vi "ArmSimulator.vi"() -> ()   [LabVIEW 2020]
uses:
  <vilib>/robotics/Kinematics/DH Kinematic Parameters.ctl
  <vilib>/robotics/Kinematics/Link/Joint Type.ctl
  <vilib>/Utility/miscctls.llb/LV3DPointTypeDef.ctl
  de8be538-574b-4146-99e0-83cb54bb3f19.vi
  a5137bdd-6b26-409e-be81-2a36b3426dbb.vi
  <vilib>/robotics/Kinematics/RotateX.vi
  <vilib>/robotics/Kinematics/RotateY.vi
  <vilib>/robotics/Kinematics/RotateZ.vi
  <vilib>/Analysis/baseanly.llb/A x B.vi
  <vilib>/Analysis/baseanly.llb/Real A x B.vi
  <vilib>/robotics/Kinematics/Analytical/Initialize Generic Serial Arm.vi
  <vilib>/robotics/Kinematics/Robot/Forward Kinematics (Point).vi
  <vilib>/picture/3D Picture Control/Object/Create Object (drawable).vi
  <vilib>/Analysis/Matrix/Comparison/Not Equal/Not Equal.vi
  <vilib>/Analysis/Matrix/Comparison/Not Equal/Not Equal - RM,RM.vi
  <vilib>/picture/3D Picture Control/Object/Add Object (no reference).vi
  <vilib>/robotics/Kinematics/Analytical/NI_Robotics_AnalyticKinematics.lvlib
  <vilib>/robotics/Kinematics/Link/NI_Robotics_Link.lvclass
  <vilib>/robotics/Kinematics/Robot/NI_Robotics_Serial Robot Arm.lvclass
  <vilib>/robotics/Kinematics/Plotting/NI_Robotics_3DKinematics.lvlib
  <vilib>/picture/3D Picture Control/NI_3D Picture Control.lvlib
  <vilib>/robotics/Kinematics/NI_Kinematics.lvlib
panel:
  in  "Wrist Position":bool
  out "Steps Taken":i32
  in  "Reset 3D View":bool
  out "IK Error":errorcluster
  in  "Goal Z (in)":dbl=28.0
  in  "Goal X (in)":dbl=-33.0
  out "3D Arm Simulation":refnum<vi>(3d-picture)
  # "<-- DOWN FIELD              SCORING GRID -->"
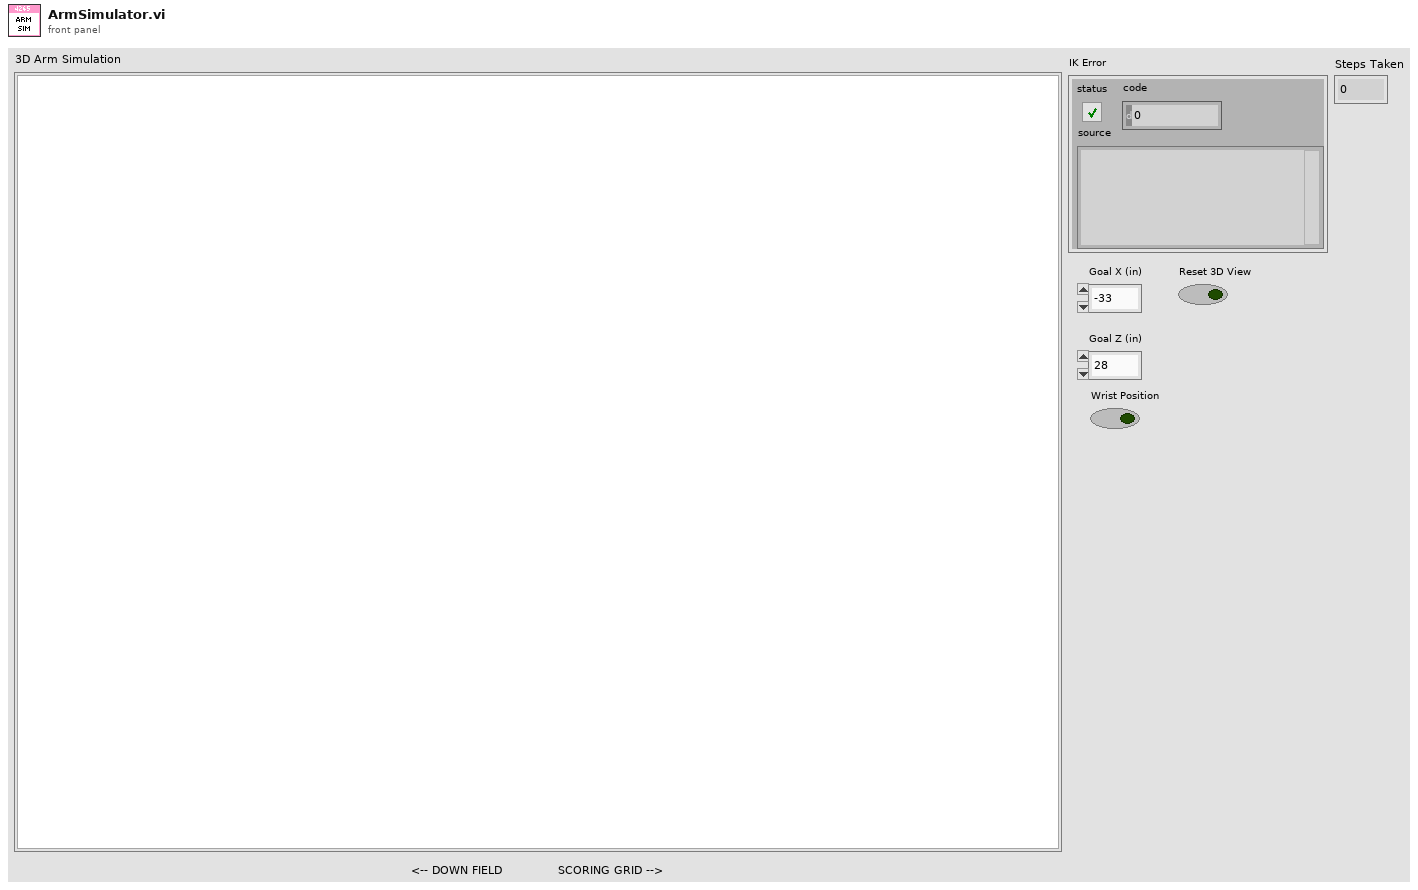
[diagram p1: front panel]
types:
  T1 = typedef "DH Kinematic Parameters.ctl" = cluster{"twist angle":dbl, "length":dbl, "rotation angle":dbl, "offset distance":dbl, "joint type":T2, "joint coordinate offset":dbl}
  T2 = typedef "NI_Robotics_Link.lvclass/Joint Type.ctl" = enum16{"Revolute", "Prismatic"}
  T3 = typedef "NI_Matrix.lvlib/RealMatrix.ctl" = dbl[][]
  T4 = cluster{"Red":sgl, "Green":sgl, "Blue":sgl, "Alpha":sgl}
  T5 = typedef "LV3DPointTypeDef.ctl" = cluster{"X":sgl, "Y":sgl, "Z":sgl}
  T6 = cluster{"Goal X (in)":dbl, "Goal Y (in)":dbl, "Goal Z (in)":dbl}
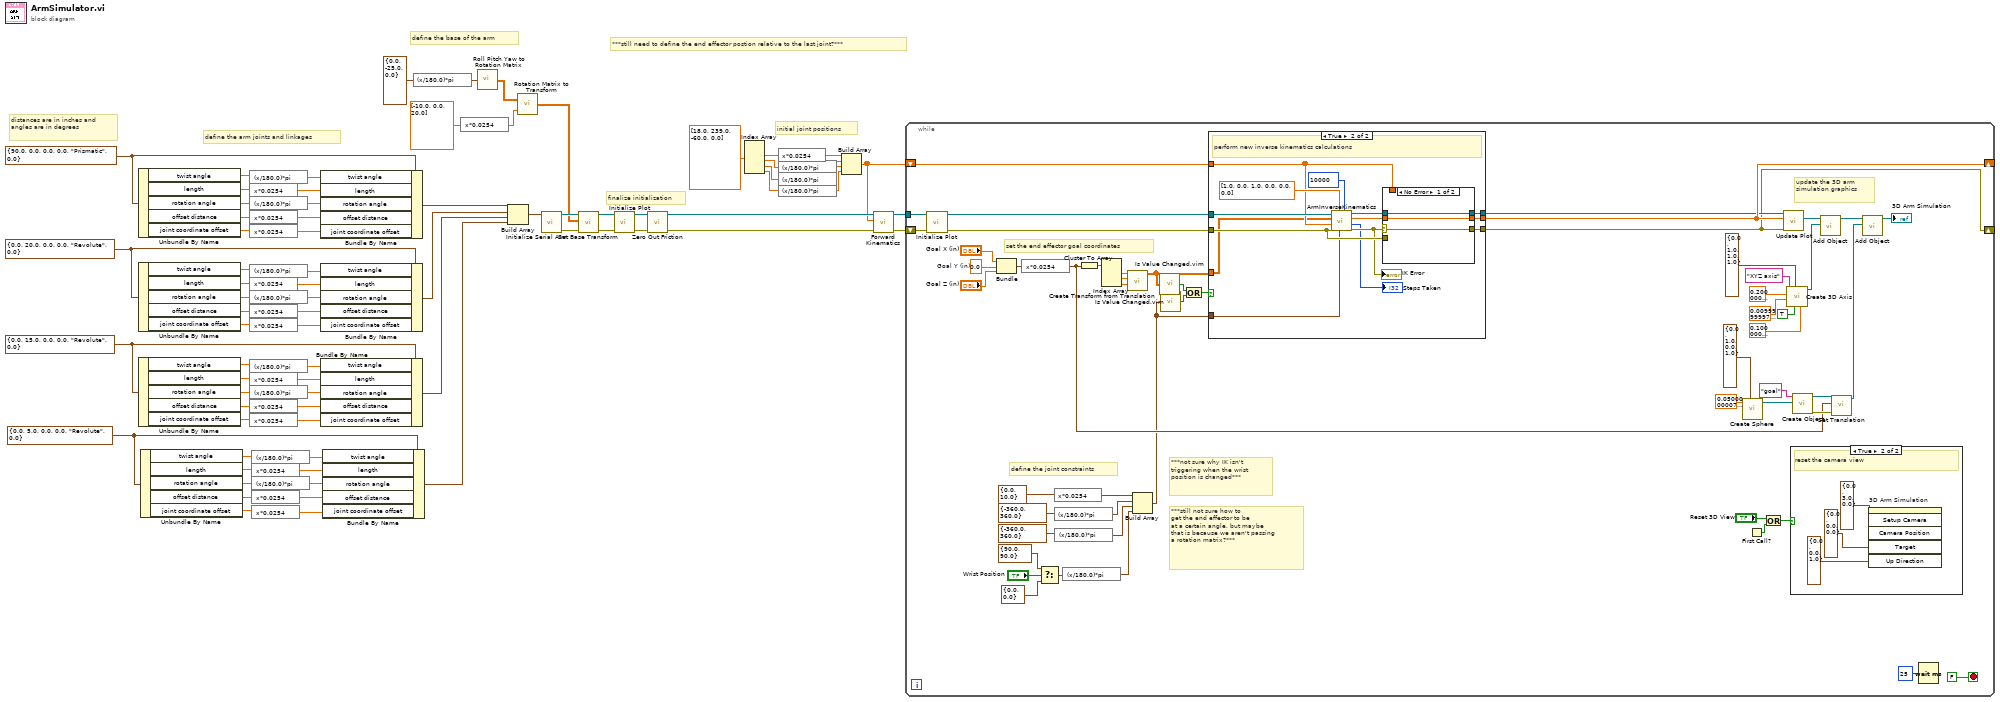
[diagram p0: block diagram]
diagram:
  w13 = T1 {"twist angle"=0.0, "length"=5.0, "rotation angle"=0.0, "offset distance"=0.0, "joint type"=enum."Revolute", "joint coordinate offset"=0.0} ("Link Parameters")
  w49 = T1 {"twist angle"=0.0, "length"=15.0, "rotation angle"=0.0, "offset distance"=0.0, "joint type"=enum."Revolute", "joint coordinate offset"=0.0} ("Link Parameters")
  w60 = T1 {"twist angle"=0.0, "length"=20.0, "rotation angle"=0.0, "offset distance"=0.0, "joint type"=enum."Revolute", "joint coordinate offset"=0.0} ("Link Parameters")
  w72 = T1 {"twist angle"=90.0, "length"=0.0, "rotation angle"=0.0, "offset distance"=0.0, "joint type"=enum."Prismatic", "joint coordinate offset"=0.0} ("Link Parameters")
  # "***still need to define the end effector postion relative to the last joint?***"
  # "initial joint positions"
  # "define the arm joints and linkages"
  # "define the base of the arm"
  # "distances are in inches and\nangles are in degrees"
  # "finalize initialization"
  n1 = Unbundle By Name(w72) -> ("twist angle"=w71:dbl, "length"=w67:dbl, "rotation angle"=w69:dbl, "offset distance"=w65:dbl, "joint coordinate offset"=w63:dbl)
  n2 = Unbundle By Name(w60) -> ("twist angle"=w59:dbl, "length"=w56:dbl, "rotation angle"=w58:dbl, "offset distance"=w54:dbl, "joint coordinate offset"=w52:dbl)
  n3 = Unbundle By Name(w49) -> ("twist angle"=w48:dbl, "length"=w45:dbl, "rotation angle"=w47:dbl, "offset distance"=w43:dbl, "joint coordinate offset"=w41:dbl)
  n4 = Unbundle By Name(w13) -> ("twist angle"=w12:dbl, "length"=w9:dbl, "rotation angle"=w11:dbl, "offset distance"=w7:dbl, "joint coordinate offset"=w5:dbl)
  n5 = expression code="(x/180.0)*pi" ("degrees to radians")(w71) -> (w73:dbl)
  n6 = expression code="x*0.0254" ("degrees to radians")(w67) -> (w66:dbl)
  n7 = expression code="(x/180.0)*pi" ("degrees to radians")(w69) -> (w68:dbl)
  n8 = expression code="x*0.0254" ("degrees to radians")(w65) -> (w64:dbl)
  n9 = expression code="x*0.0254" ("degrees to radians")(w63) -> (w62:dbl)
  n10 = expression code="(x/180.0)*pi" ("degrees to radians")(w59) -> (w61:dbl)
  n11 = expression code="x*0.0254" ("degrees to radians")(w56) -> (w55:dbl)
  n12 = expression code="(x/180.0)*pi" ("degrees to radians")(w58) -> (w57:dbl)
  n13 = expression code="x*0.0254" ("degrees to radians")(w54) -> (w53:dbl)
  n14 = expression code="x*0.0254" ("degrees to radians")(w52) -> (w51:dbl)
  n15 = expression code="(x/180.0)*pi" ("degrees to radians")(w48) -> (w50:dbl)
  n16 = expression code="x*0.0254" ("degrees to radians")(w45) -> (w44:dbl)
  n17 = expression code="(x/180.0)*pi" ("degrees to radians")(w47) -> (w46:dbl)
  n18 = expression code="x*0.0254" ("degrees to radians")(w43) -> (w42:dbl)
  n19 = expression code="x*0.0254" ("degrees to radians")(w41) -> (w40:dbl)
  n20 = expression code="(x/180.0)*pi" ("degrees to radians")(w12) -> (w14:dbl)
  n21 = expression code="x*0.0254" ("degrees to radians")(w9) -> (w8:dbl)
  n22 = expression code="(x/180.0)*pi" ("degrees to radians")(w11) -> (w10:dbl)
  n23 = expression code="x*0.0254" ("degrees to radians")(w7) -> (w6:dbl)
  n24 = expression code="x*0.0254" ("degrees to radians")(w5) -> (w4:dbl)
  n25 = Bundle By Name(cluster=w72, "twist angle"=w73, "length"=w66, "rotation angle"=w68, "offset distance"=w64, "joint coordinate offset"=w62) -> (w70:T1)
  n26 = Bundle By Name(cluster=w60, "twist angle"=w61, "length"=w55, "rotation angle"=w57, "offset distance"=w53, "joint coordinate offset"=w51) -> (w39:T1)
  n27 = Bundle By Name(cluster=w49, "twist angle"=w50, "length"=w44, "rotation angle"=w46, "offset distance"=w42, "joint coordinate offset"=w40) -> (w38:T1)
  n28 = Bundle By Name(cluster=w13, "twist angle"=w14, "length"=w8, "rotation angle"=w10, "offset distance"=w6, "joint coordinate offset"=w4) -> (w3:T1)
  n29 = expression code="(x/180.0)*pi" ("degrees to radians")(cluster{"roll":dbl, "pitch":dbl, "yaw":dbl} {"roll"=0.0, "pitch"=-25.0, "yaw"=0.0} ("angles")) -> (w33:cluster{"roll":dbl, "pitch":dbl, "yaw":dbl})
  n30 = expression code="x*0.0254" ("degrees to radians")(dbl[] [-10.0, 0.0, 20.0] ("translation vector")) -> (w28:dbl[])
  n31 = call <vilib>:"Roll Pitch Yaw to Rotation Matrix.vi"("angles"=w33) -> ("rotation matrix"=w35:T3)
  n32 = Build Array(w70, w39, w38, w3) -> (w37:T1[])
  n33 = call <vilib>:"Rotation Matrix to Transform.vi"("translation vector"=w28, "rotation matrix"=w35) -> ("transform"=w32:T3)
  n34 = call-poly <vilib>:"Initialize Serial Arm.vi"("kinematic parameters"=w37) -> ("error out"=w30:errorcluster, "serial arm out"=w36:refnum<class "NI_Robotics_Serial Robot Arm.lvclass">)  [unwired: 9 in]
  n35 = call <vilib>:"Set Base Transform.vi"("error in (no error)"=w30, "base transform"=w32, "serial arm in"=w36) -> ("error out"=w29:errorcluster, "serial arm out"=w31:refnum<class "NI_Robotics_Serial Robot Arm.lvclass">)  [unwired: 7 in]
  n36 = call <vilib>:"Initialize Plot.vi"("error in (no error)"=w29, "serial arm in"=w31) -> ("error out"=w75:errorcluster, "serial arm out"=w74:refnum<class "NI_Robotics_Serial Robot Arm.lvclass">)  [unwired: 8 in]
  n37 = call <vilib>:"Zero Out Friction.vi"("error in (no error)"=w75, "serial arm in"=w74) -> ("error out"=w18:errorcluster, "serial arm out"=w19:refnum<class "NI_Robotics_Serial Robot Arm.lvclass">)  [unwired: 8 in]
  n38 = Index Array(array=dbl[] [18.0, 239.0, -60.0, 0.0] ("Joint Positions 2")) -> (element #1=w21:dbl, element #2=w23:dbl, element #3=w25:dbl, element #4=w2:dbl)  [unwired: 4 in]
  n39 = expression code="x*0.0254" ("degrees to radians")(w21) -> (w20:dbl)
  n40 = expression code="(x/180.0)*pi" ("degrees to radians")(w23) -> (w22:dbl)
  n41 = expression code="(x/180.0)*pi" ("degrees to radians")(w25) -> (w24:dbl)
  n42 = expression code="(x/180.0)*pi" ("degrees to radians")(w2) -> (w1:dbl)
  n43 = Build Array(w20, w22, w24, w1) -> (w15:dbl[])
  n44 = call-poly <vilib>:"Forward Kinematics.vi"("error in (no error)"=w18, "joint positions"=w15, "serial arm in"=w19) -> ("error out"=w16:errorcluster, "serial arm out"=w17:refnum<class "NI_Robotics_Serial Robot Arm.lvclass">)  [unwired: 6 in, 1 out]
  n45 = while {
    tunnel: w17 -> [w114]
    shift-right: [w107] -> _
    shift-left: w15 -> [w94]
    shift-right: [w91] -> _
    shift-left: w16 -> [w113]
    stop <- FALSE stop-if-true
    w109 = 0.0  # Goal Y (in)
    # "***still not sure how to\nget the end effector to be\nat a certain angle, but maybe \nthat is because we aren't passing\na rotation matrix?***"
    # "***not sure why IK isn't\ntriggering when the wrist\nposition is changed***"
    # "define the joint constraints"
    # "set the end effector goal coordinates"
    # "update the 3D arm\nsimulation graphics"
    n46 = call <vilib>:"Initialize Plot.vi"("error in (no error)"=w113, "serial arm in"=w114) -> ("error out"=w105:errorcluster, "serial arm out"=w102:refnum<class "NI_Robotics_Serial Robot Arm.lvclass">)  [unwired: 8 in]
    n47 = Bundle("Goal X (in)"="Goal X (in)", "Goal Y (in)"=w109, "Goal Z (in)"="Goal Z (in)") -> (w104:T6)  [unwired: 1 in]
    n48 = expression code="x*0.0254" ("degrees to radians")(w104) -> (w103:T6)
    n49 = Select(t=cluster{dbl, dbl} {90.0, 90.0}, s="Wrist Position", f=cluster{dbl, dbl} {0.0, 0.0}) -> (s? t:f=w77:cluster{dbl, dbl})
    n50 = expression code="x*0.0254" ("degrees to radians")(cluster{dbl, dbl} {0.0, 10.0}) -> (w90:cluster{dbl, dbl})
    n51 = expression code="(x/180.0)*pi" ("degrees to radians")(cluster{dbl, dbl} {-360.0, 360.0}) -> (w80:cluster{dbl, dbl})
    n52 = expression code="(x/180.0)*pi" ("degrees to radians")(cluster{dbl, dbl} {-360.0, 360.0}) -> (w78:cluster{dbl, dbl})
    n53 = expression code="(x/180.0)*pi" ("degrees to radians")(w77) -> (w76:cluster{dbl, dbl})
    n54 = Cluster To Array(cluster=w103) -> (array=w93:dbl[])
    n55 = Index Array(array=w93) -> (element #1=w97:dbl, element #2=w96:dbl, element #3=w95:dbl)  [unwired: 3 in]
    n56 = call <vilib>:"Create Transform from Translation.vi"("z"=w95, "y"=w96, "x"=w97) -> ("transform"=w92:T3)  [unwired: 8 in]
    n57 = Build Array(w90, w80, w78, w76) -> (w86:cluster{dbl, dbl}[])
    n58 = call "Is Value Changed.vim"("value"=w92) -> ("changed or first call?"=w83:bool)
    n59 = call "Is Value Changed.vim"("value"=w86) -> ("changed or first call?"=w84:bool)
    n60 = Compound Arithmetic op=OR(w83, w84) -> (w85:bool)
    n61 = case shown="True" w85 {
      tunnel: [w131 w145] -> w107
      tunnel: [w133 w143] -> w106
      tunnel: [w132 w142] -> w91
      tunnel: w105 -> [w132 w141]
      tunnel: w102 -> [w133 w139]
      tunnel: w94 -> [w131 w137]
      tunnel: w86 -> [_ w136]
      tunnel: w92 -> [_ w135]
      frame False {
        # "the end effector goal postion has not changed"
      }
      frame True {
        # "perform new inverse kinematics calculations"
        n62 = call "ArmInverseKinematics.vi"("max steps"=10000, "joint constraints"=w136, "mask"=dbl[] [1.0, 0.0, 1.0, 0.0, 0.0, 0.0], "error in (no error)"=w141, "current joint positions"=w137, "end effector transform"=w135, "serial arm in"=w139) -> ("error out"=w140:errorcluster, "steps taken"=→"Steps Taken":i32, "joint positions"=w146:dbl[], "serial arm out"=w144:refnum<class "NI_Robotics_Serial Robot Arm.lvclass">)  [unwired: 1 in]
        "IK Error" <- w140
        n63 = case shown="No Error" w140 {
          selector: w140 -> [w148 _]
          tunnel: w146 -> [w150 _]
          tunnel: [w150 w153] -> w145
          tunnel: w144 -> [w149 w152]
          tunnel: [w149 w152] -> w143
          tunnel: w137 -> [_ w153]
          tunnel: [w148 w151] -> w142
          tunnel: w141 -> [_ w151]
          frame No Error {
          }
          frame Error {
          }
        }
      }
    }
    n64 = call <vilib>:"Create Sphere.vi"("Color"=T4 {"Red"=0.0, "Green"=1.0, "Blue"=0.0, "Alpha"=1.0}, "Radius"=sgl 0.05) -> ("New Sphere Refnum"=w110:refnum<vi>)  [unwired: 8 in, 1 out]
    n65 = First Call?() -> (First Call?: T/F=w101:bool)
    n66 = Or(x="Reset 3D View", y=w101) -> (x .or. y?=w100:bool)
    n67 = call <vilib>:"Update Plot.vi"("error in (no error)"=w91, "joint positions"=w107, "serial arm in"=w106) -> ("serial arm scene"=w128:refnum<vi>)  [unwired: 6 in, 2 out]
    n68 = call <vilib>:"Create 3D Axis.vi"("Character Size"=sgl 0.1, "Axis label?"=TRUE, "Color"=T4 {"Red"=0.0, "Green"=1.0, "Blue"=1.0, "Alpha"=1.0}, "Radius"=sgl 0.01, "Length"=sgl 0.2, "Name"="XYZ axis") -> ("New Object Refnum"=w121:refnum<vi>)  [unwired: 4 in, 1 out]
    n69 = case shown="True" w100 {
      frame False {
      }
      frame True {
        # "reset the camera view"
        n70 = invoke on="3D Arm Simulation" class="SceneGraphDisp (strict)" method="Setup Camera"("Camera Position"=T5 {"X"=0.0, "Y"=3.0, "Z"=0.0}, "Target"=T5 {"X"=0.0, "Y"=0.0, "Z"=0.0}, "Up Direction"=T5 {"X"=0.0, "Y"=0.0, "Z"=1.0}) -> ()  [unwired: 3 in, 6 out]
      }
    }
    n71 = call-poly <vilib>:"Create Object.vi"("Geometry"=w110, "Name"="goal") -> ("error out"=w118:errorcluster, "Scene:New Object"=w115:refnum<vi>)  [unwired: 8 in]
    n72 = call-poly <vilib>:"Add Object.vi"("New Object In"=w121, "Scene Object In"=w128) -> ("Scene Object Out"=w120:refnum<vi>)  [unwired: 8 in, 1 out]
    n73 = call <vilib>:"Set Translation.vi"("error in (no error)"=w118, "Translation"=w103, "Scene Object"=w115) -> ("Translated Object"=w119:refnum<vi>)  [unwired: 7 in, 1 out]
    n74 = call-poly <vilib>:"Add Object.vi"("New Object In"=w119, "Scene Object In"=w120) -> ("Scene Object Out"=→"3D Arm Simulation":refnum<vi>)  [unwired: 8 in, 1 out]
    n75 = Wait (ms)(milliseconds to wait=u32 25) -> ()  [unwired: 1 out]
  }
